vi "Maxi Gauge-Test Display,Memory.vi"(8 "Fehler (Eingang)":errorcluster, 9 "Testfunction":u8(ring) items=["Display Test", "EEPROM Test", "EPROM Test", "RAM Test"], 10 "Node address":i8=-1 min=-1 max=31 step=1, 11 "VISA-Ressource in":refnum<visa-resource-name>) -> (0 "Fehler (Ausgang)":errorcluster, 1 "Sensor Errorstatus":u16, 2 "Gauge Errorstatus":u16, 3 "VISA-Ressource out":refnum<visa-resource-name>, 4 "Errortext":string[](array[string]))   [LabVIEW 2012, in "Maxi Gauge.lvlib"]
uses:
  Maxi Gauge.lvlib
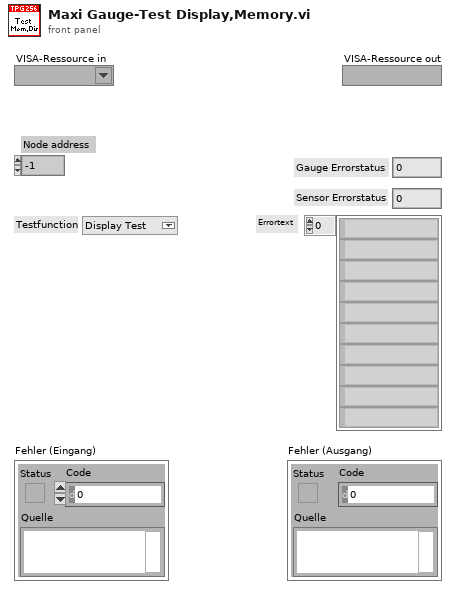
[diagram p1: front panel]
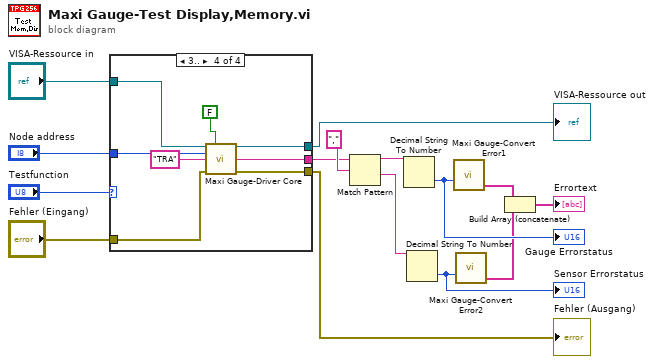
[diagram p0: block diagram]
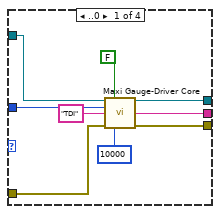
[diagram p2: hidden frame]
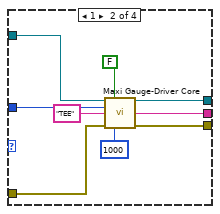
[diagram p3: hidden frame]
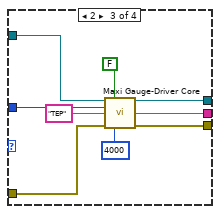
[diagram p4: hidden frame]
diagram:
  n1 = case shown="3.." "Testfunction" {
    tunnel: "Node address" -> [w24 w33 w42 w50]
    tunnel: [w23 w31 w39 w47] -> w5
    tunnel: [w20 w28 w40 w48] -> w3
    tunnel: "Fehler (Eingang)" -> [w18 w25 w34 w43]
    tunnel: "VISA-Ressource in" -> [w17 w26 w35 w44]
    tunnel: [w16 w27 w36 w45] -> w1
    frame ..0 {
      n2 = call "Maxi Gauge-Driver Core.vi"("VISA-Ressource in"=w17, "Write/Read"=FALSE, "Node address"=w24, "Command"="TDI", "Fehler (Eingang)"=w18, "Timeout [ms]"=u32 10000) -> ("VISA-Ressource out"=w16:refnum<visa-resource-name>, "String Out"=w23:string, "Fehler (Ausgang)"=w20:errorcluster)  [unwired: 7 in]
    }
    frame 1 {
      n3 = call "Maxi Gauge-Driver Core.vi"("VISA-Ressource in"=w26, "Write/Read"=FALSE, "Node address"=w33, "Command"="TEE", "Fehler (Eingang)"=w25, "Timeout [ms]"=u32 1000) -> ("VISA-Ressource out"=w27:refnum<visa-resource-name>, "String Out"=w31:string, "Fehler (Ausgang)"=w28:errorcluster)  [unwired: 7 in]
    }
    frame 2 {
      n4 = call "Maxi Gauge-Driver Core.vi"("VISA-Ressource in"=w35, "Write/Read"=FALSE, "Node address"=w42, "Command"="TEP", "Fehler (Eingang)"=w34, "Timeout [ms]"=u32 4000) -> ("VISA-Ressource out"=w36:refnum<visa-resource-name>, "String Out"=w39:string, "Fehler (Ausgang)"=w40:errorcluster)  [unwired: 7 in]
    }
    frame 3.. {
      n5 = call "Maxi Gauge-Driver Core.vi"("VISA-Ressource in"=w44, "Write/Read"=FALSE, "Node address"=w50, "Command"="TRA", "Fehler (Eingang)"=w43) -> ("VISA-Ressource out"=w45:refnum<visa-resource-name>, "String Out"=w47:string, "Fehler (Ausgang)"=w48:errorcluster)  [unwired: 8 in]
    }
  }
  "Fehler (Ausgang)" <- w3
  "VISA-Ressource out" <- w1
  n6 = Match Pattern(string=w5, regular expression=",") -> (before substring=w9:string, after substring=w8:string)  [unwired: 1 in, 2 out]
  n7 = Decimal String To Number(string=w9) -> (number=w14:i32)  [unwired: 2 in, 1 out]
  "Gauge Errorstatus" <- w14
  n8 = Decimal String To Number(string=w8) -> (number=w12:i32)  [unwired: 2 in, 1 out]
  "Sensor Errorstatus" <- w12
  n9 = call "Maxi Gauge-Convert Error1.vi"("Errorwort1"=w14) -> ("Error Text"=w7:string[])  [unwired: 4 in]
  n10 = call "Maxi Gauge-Convert Error2.vi"("Errorwort1"=w12) -> ("Error Text"=w6:string[])  [unwired: 4 in]
  n11 = Build Array (concatenate)(w7, w6) -> (→"Errortext":string[])
